vi "PIO Read Scalar vs Array.vi"() -> ()   [LabVIEW 2016]
uses:
  <vilib>/Platform/TimedLoop/XDataNode/timing_clust.ctl
  <vilib>/Platform/TimedLoop/XDataNode/nitl_modes.ctl
  <vilib>/Platform/TimedLoop/XDataNode/wakeup.ctl
  Source/GE 5565PIORC/GE 5565PIORC Old.lvclass/GE 5565PIORC Old.ctl
  <vilib>/Instr/_visa.llb/VISA Register Access Address Space.ctl
  Source/GE 5565PIORC/VIs/Registers/Local Configuration.LAS1RR.Address Range.Get.vi
  Source/GE 5565PIORC/VIs/Registers/Local Configuration.Get Register Offset.vi
  Source/GE 5565PIORC/GE 5565PIORC Old.lvclass
  <vilib>/platform/TimedLoop/XDataNode/XDataNode.xnode
  <vilib>/Platform/TimedLoop/XDataNode/XDNodeRunTimeDep.lvlib
panel:
  in  "Iterations":i32=1000
  out "Multiple":dbl
  in  "U32 Count":i32=100
  out "Single":dbl
  in  "VISA resource name":refnum<visa-resource-name>
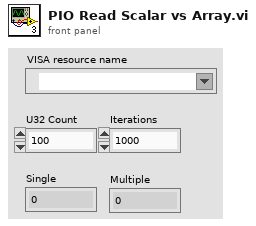
[diagram p1: front panel]
types:
  T1 = typedef "XDNodeRunTimeDep.lvlib/timing_clust.ctl" = cluster{"Expected End [f-1]":u64, "Actual End [f-1]":u64, "Finished Late? [f-1]":bool, "Expected End [i-1]":u64, "Actual End [i-1]":u64, "Finished Late? [i-1]":bool, "Expected Start [i]":u64, "Actual Start [i]":u64, "Expected Start [f]":u64, "Actual Start [f]":u64, "Source Name":string, "Structure Name":string, "Period":i64, "Deadline":i64, "Offset":i64, "Start":i64, "Priority":i32, "Timeout":i32, "Mode":T2, "Wakeup Reason":T3, "Error":errorcluster, "Source Type":string, "Secondary Source Type":string, "Global End Time":u64, "Global Start Time":u64, "Frame Duration":u64, "Iteration Duration":u64, "Assigned CPU":i32, "I/O Scan Engine Mode":u32}
  T2 = typedef "XDNodeRunTimeDep.lvlib/nitl_modes.ctl" = enum32{"No Change", "Process missed periods, maintain original phase", "Discard missed periods, maintain original phase", "Process missed periods, ignore original phase", "Discard missed periods, ignore original phase"}
  T3 = typedef "XDNodeRunTimeDep.lvlib/wakeup.ctl" = enum32{"Normal", "Aborted", "Asynchronous wakeup", "Timing source error", "Timed loop error", "Timeout"}
  T4 = typedef "VISA Register Access Address Space.ctl" = u16
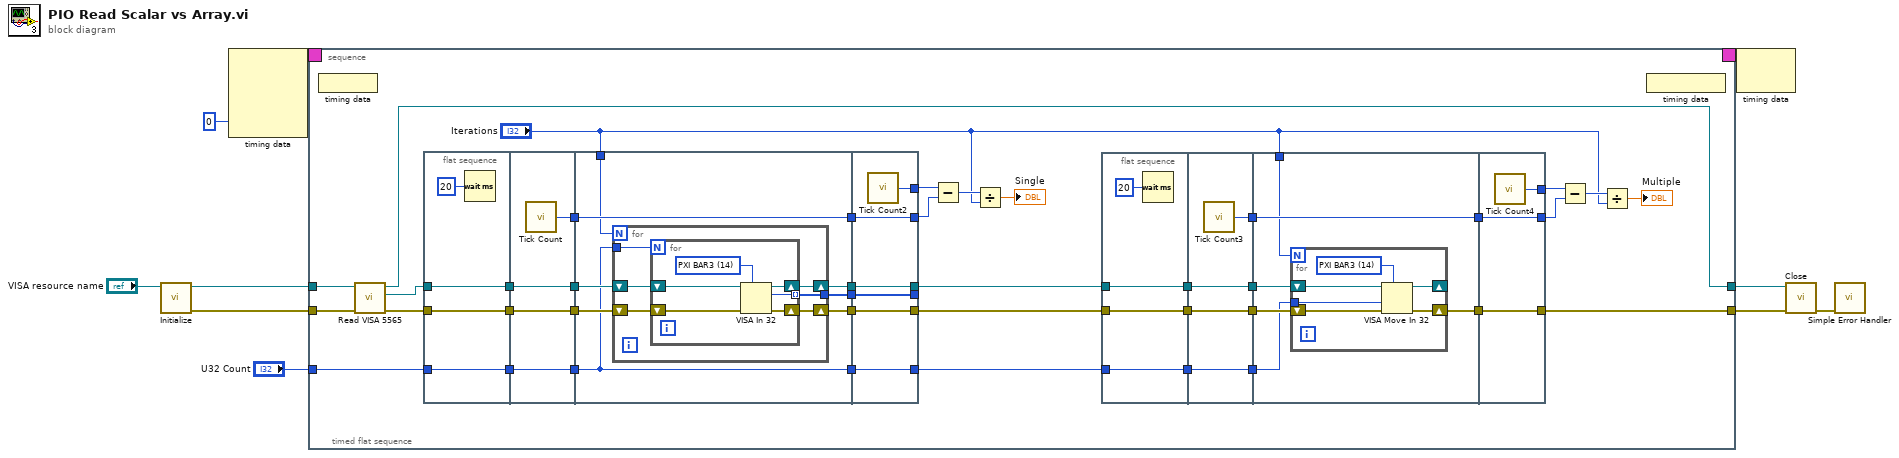
[diagram p0: block diagram]
diagram:
  n1 = call "Initialize.vi"("VISA resource name"="VISA resource name") -> ("error out"=w4:errorcluster, "GE 5565PIORC"=w5:refnum<class "GE 5565PIORC Old.lvclass">)  [unwired: 9 in]
  n2 = node-c288(0 ("Processor")) -> (w10:T1)  [unwired: 3 in]
  n3 = timed-sequence {
    timing: w10 -> [_]
    timing-out: [_] -> w9
    tunnel: w5 -> [w13]
    tunnel: w4 -> [w15]
    tunnel: "U32 Count" -> [w14]
    tunnel: [w12] -> w2
    tunnel: [w11] -> w1
    n4 = timed-flat-sequence {
      tunnel: w15 -> [w41]
      tunnel: w14 -> [w46]
      tunnel: w13 -> [w42]
      tunnel: [w18] -> w12
      tunnel: [w19] -> w11
      n5 = node-c288() -> ()  [unwired: 1 in]
      n6 = call "Read VISA 5565.vi"("error in (no error)"=w41, "GE 5565PIORC in"=w42) -> ("error out"=w40:errorcluster, "VISA 5565"=w38:refnum<visa-resource-name>, "GE 5565PIORC out"=w19:refnum<class "GE 5565PIORC Old.lvclass">)  [unwired: 7 in]
      n7 = flat-sequence {
        tunnel: w40 -> [w81]
        tunnel: [w81] -> w50
        tunnel: w46 -> [w80]
        tunnel: [w80] -> w45
        tunnel: w38 -> [w79]
        tunnel: [w79] -> w37
        tunnel: [w86] -> w55
        tunnel: [w85] -> w51
        tunnel: w50 -> [w85]
        tunnel: w45 -> [w84]
        tunnel: [w84] -> w44
        tunnel: [w83] -> w39
        tunnel: w37 -> [w83]
        tunnel: w55 -> [w94]
        tunnel: [w94] -> w54
        tunnel: w51 -> [w92]
        tunnel: [w93] -> w49
        tunnel: w44 -> [w88]
        tunnel: [w88] -> w43
        tunnel: w39 -> [w91]
        tunnel: [w90] -> w36
        tunnel: "Iterations" -> [w89]
        tunnel: [w87] -> w17
        tunnel: [w112] -> w53
        tunnel: [w111] -> w52
        tunnel: w54 -> [w111]
        tunnel: w49 -> [w108]
        tunnel: [w108] -> w16
        tunnel: w43 -> [w110]
        tunnel: [w110] -> w21
        tunnel: w36 -> [w109]
        tunnel: [w109] -> w22
        tunnel: w17 -> [w107]
        tunnel: [w107] -> _
        frame #0 {
          n8 = Wait (ms)(milliseconds to wait=u32 20) -> ()  [unwired: 1 out]
        }
        frame #1 {
          n9 = call "Tick Count"() -> ("Tick Count(uSec)"=w86:u32)
        }
        frame #2 {
          n10 = for {
            N: w89 -> [_]
            shift-right: [w97] -> w93
            shift-left: w92 -> [w98]
            shift-right: [w99] -> w90
            shift-left: w91 -> [w100]
            tunnel: w88 -> [w95]
            tunnel: [w96] -> w87
            n11 = for {
              N: w95 -> [_]
              shift-right: [w105] -> w99
              shift-left: w100 -> [w106]
              shift-right: [w103] -> w97
              shift-left: w98 -> [w104]
              tunnel: [w101] -> w96 mode=indexing
              w102 = T4 14 items=["VXI/VME A16"=1, "VXI/VME A24"=2, "VXI/VME A32"=3, "VXI/VME A64"=4, "PXI Memory Allocations"=9, "PXI Configuration"=10, "PXI BAR0"=11, "PXI BAR1"=12, "PXI BAR2"=13, "PXI BAR3"=14, "PXI BAR4"=15, "PXI BAR5"=16] ("Address Space")
              n12 = VISA In 32(7:w102, 8:w104, 11:w106) -> (0:w103:errorcluster, 2:w101:u32, 3:w105:refnum<visa-resource-name>)  [unwired: 1 in]
            }
          }
        }
        frame #3 {
          n13 = call "Tick Count2"() -> ("Tick Count(uSec)"=w112:u32)
        }
      }
      n14 = Subtract(x=w53, y=w52) -> (x-y=w48:u32)
      n15 = Divide(x=w48, y="Iterations") -> (x/y=→"Single":dbl)
      n16 = flat-sequence {
        tunnel: w16 -> [w58]
        tunnel: [w58] -> w35
        tunnel: w21 -> [w57]
        tunnel: [w57] -> w34
        tunnel: w22 -> [w56]
        tunnel: [w56] -> w33
        tunnel: [w63] -> w32
        tunnel: [w62] -> w31
        tunnel: w35 -> [w62]
        tunnel: w34 -> [w61]
        tunnel: [w61] -> w30
        tunnel: [w60] -> w29
        tunnel: w33 -> [w60]
        tunnel: w32 -> [w69]
        tunnel: [w69] -> w28
        tunnel: w31 -> [w67]
        tunnel: [w68] -> w27
        tunnel: w30 -> [w64]
        tunnel: w29 -> [w66]
        tunnel: "Iterations" -> [w65]
        tunnel: [w78] -> w26
        tunnel: [w77] -> w25
        tunnel: w28 -> [w77]
        tunnel: w27 -> [w76]
        tunnel: [w76] -> w18
        frame #0 {
          n17 = Wait (ms)(milliseconds to wait=u32 20) -> ()  [unwired: 1 out]
        }
        frame #1 {
          n18 = call "Tick Count3"() -> ("Tick Count(uSec)"=w63:u32)
        }
        frame #2 {
          n19 = for {
            N: w65 -> [_]
            shift-right: [w72] -> w68
            shift-left: w67 -> [w73]
            shift-right: [w74] -> _
            shift-left: w66 -> [w75]
            tunnel: w64 -> [w70]
            w71 = T4 14 items=["VXI/VME A16"=1, "VXI/VME A24"=2, "VXI/VME A32"=3, "VXI/VME A64"=4, "PXI Memory Allocations"=9, "PXI Configuration"=10, "PXI BAR0"=11, "PXI BAR1"=12, "PXI BAR2"=13, "PXI BAR3"=14, "PXI BAR4"=15, "PXI BAR5"=16] ("Address Space")
            n20 = VISA Move In 32(7:w71, 8:w73, 9:w70, 11:w75) -> (0:w72:errorcluster, 3:w74:refnum<visa-resource-name>)  [unwired: 1 in, 1 out]
          }
        }
        frame #3 {
          n21 = call "Tick Count4"() -> ("Tick Count(uSec)"=w78:u32)
        }
      }
      n22 = Subtract(x=w26, y=w25) -> (x-y=w24:u32)
      n23 = Divide(x=w24, y="Iterations") -> (x/y=→"Multiple":dbl)
      n24 = node-c288() -> ()  [unwired: 1 out]
    }
  }
  n25 = node-c288(w9) -> ()  [unwired: 1 out]
  n26 = call "Close.vi"("error in (no error)"=w2, "GE 5565PIORC in"=w1) -> ("error out"=w7:errorcluster)  [unwired: 8 in, 1 out]
  n27 = call <vilib>:"Simple Error Handler.vi"("error in (no error)"=w7) -> ()  [unwired: 4 in, 5 out]
